vi "Check to Close.vi"(8 "error in (no error)":errorcluster, 11 "Messaging Server Module in":refnum<class "Messaging Server Module.lvclass">) -> (0 "error out":errorcluster, 3 "Messaging Server Module out":refnum<class "Messaging Server Module.lvclass">)   [LabVIEW 2020, in "Volatus.lvlib" / "Messaging Server Module.lvclass"]
uses:
  Messaging Server Module.lvclass
  Messaging Server Module.lvclass/Messaging Server Module.ctl
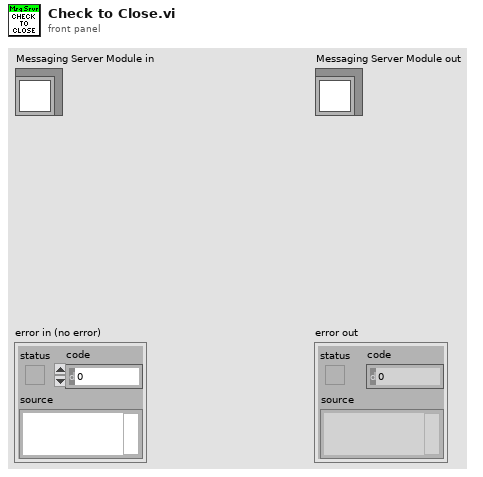
[diagram p1: front panel]
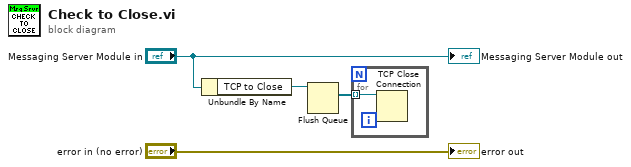
[diagram p0: block diagram]
diagram:
  n1 = Unbundle By Name("Messaging Server Module in") -> ("TCP to Close"=w2:refnum<queue>)
  n2 = Flush Queue(queue=w2) -> (remaining elements=w1:refnum<k5>[])  [unwired: 1 in, 2 out]
  n3 = for {
    tunnel: w1 -> [w5] mode=indexing
    n4 = TCP Close Connection(connection ID=w5) -> ()  [unwired: 2 in, 2 out]
  }
  "error out" <- "error in (no error)"
  "Messaging Server Module out" <- "Messaging Server Module in"
